vi "_test FollowMouse.vi"() -> ()   [LabVIEW 2013]
uses:
  Engine/Move Speed.ctl
  Engine/Positioning Strategy.ctl
panel:
  in  "Positioning Strategy":T1
  in  "Follow? (F1)":bool
  in  "Move Speed (Normal)":T2
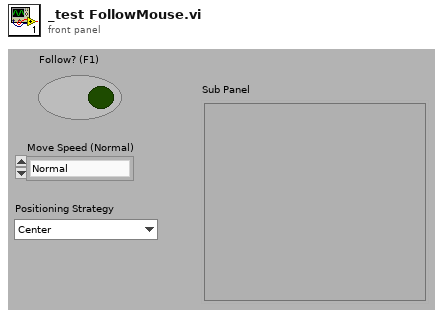
[diagram p1: front panel]
types:
  T1 = typedef "Positioning Strategy.ctl" = enum16{"Center", "Origin (Top-Left)"}
  T2 = typedef "Move Speed.ctl" = enum16{"Normal", "Fast", "Slow", "Instantaneous"}
  T3 = typedef "LVPoint32TypeDef.ctl" = cluster{"Horizontal":i32, "Vertical":i32}
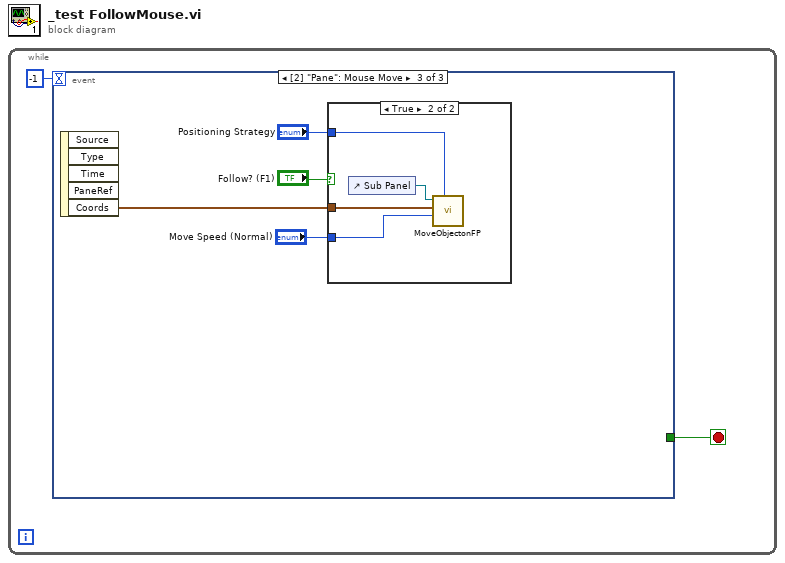
[diagram p0: block diagram]
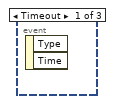
[diagram p2: hidden frame]
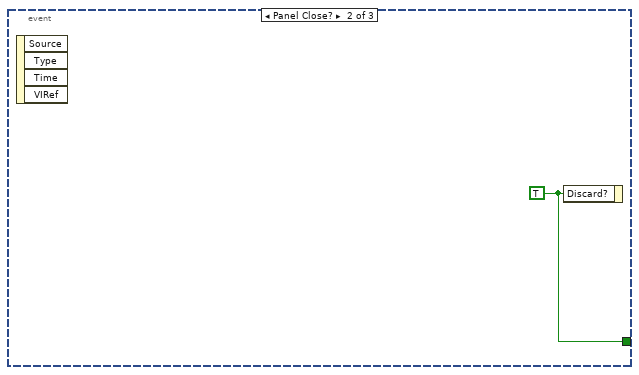
[diagram p3: hidden frame]
diagram:
  n1 = while {
    stop <- w1 stop-if-true
    n2 = event shown="[2] \"Pane\": Mouse Move" {
      selector: _ -> [_ _ _]
      dyn-events: _ -> [_ _ _]
      timeout: -1 -> [_ _ _]
      tunnel: [_ w3 _] -> w1
      event Timeout {
        n3 = event-data() -> ()  [unwired: 3 out]
      }
      event Panel Close? {
        w3 = TRUE ("Discard?")
        n4 = event-data() -> ()  [unwired: 5 out]
        n5 = event-data("Discard?"=w3) -> ()  [unwired: 1 in, 1 out]
      }
      event Mouse Move {
        n6 = event-data() -> ("Coords"=w7:T3)  [unwired: 5 out]
        n7 = case shown="True" "Follow? (F1)" {
          tunnel: w7 -> [_ w11]
          tunnel: "Move Speed (Normal)" -> [_ w10]
          tunnel: "Positioning Strategy" -> [_ w8]
          frame False {
          }
          frame True {
            n8 = control-ref of="Sub Panel"() -> (w9:refnum<vi>)
            n9 = call "MoveObjectonFP.vi"("Positioning Strategy (Center)"=w8, "Move Speed (Instantaneous)"=w10, "Center Position for Object"=w11, "GObject"=w9) -> ()  [unwired: 2 in, 6 out]
          }
        }
      }
    }
  }
